vi "RGBtoCMYK.vi"(2 "RGB in":dbl[](array[numeric]), 3 "CMYK in":dbl[](array[numeric])) -> (0 "RGB out":dbl[](array[numeric]), 1 "CMYK out":dbl[](array[numeric]))   [LabVIEW 2013]
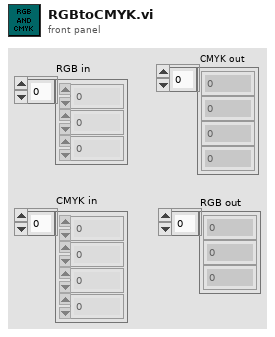
[diagram p1: front panel]
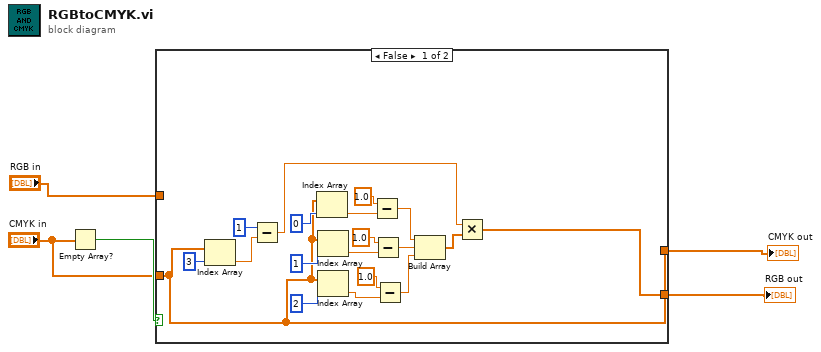
[diagram p0: block diagram]
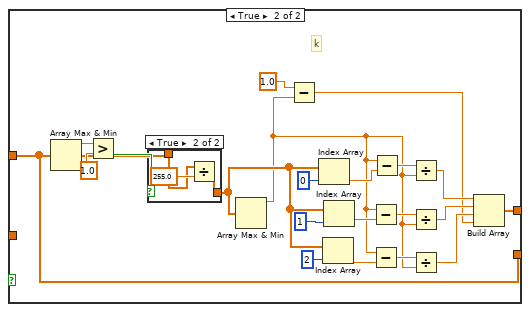
[diagram p2: hidden frame]
diagram:
  n1 = Empty Array?(array="CMYK in") -> (empty?=w4:bool)
  n2 = case shown="False" w4 {
    tunnel: "RGB in" -> [_ w25]
    tunnel: [w18 w26] -> w5
    tunnel: "CMYK in" -> [w18 _]
    tunnel: [w6 w25] -> w1
    frame False {
      n3 = Index Array(array=w18, index=3) -> (element=w23:dbl)
      n4 = Subtract(x=1, y=w23) -> (x-y=w7:dbl)
      n5 = Index Array(array=w18, index=0) -> (element=w14:dbl)
      n6 = Index Array(array=w18, index=1) -> (element=w13:dbl)
      n7 = Index Array(array=w18, index=2) -> (element=w12:dbl)
      n8 = Subtract(x=1.0, y=w14) -> (x-y=w11:dbl)
      n9 = Subtract(x=1.0, y=w13) -> (x-y=w10:dbl)
      n10 = Subtract(x=1.0, y=w12) -> (x-y=w9:dbl)
      n11 = Build Array(w11, w10, w9) -> (w8:dbl[])
      n12 = Multiply(x=w7, y=w8) -> (x*y=w6:dbl[])
    }
    frame True {
      # "k"
      n13 = Array Max & Min(array=w25) -> (max value=w32:dbl)  [unwired: 3 out]
      n14 = Greater?(x=w32, y=1.0) -> (0:w30:bool)
      n15 = case shown="True" w30 {
        tunnel: w25 -> [w46 w48]
        tunnel: [w46 w47] -> w29
        frame False {
        }
        frame True {
          n16 = Divide(x=w48, y=255.0) -> (x/y=w47:dbl[])
        }
      }
      n17 = Array Max & Min(array=w29) -> (max value=w27:dbl)  [unwired: 3 out]
      n18 = Subtract(x=1.0, y=w27) -> (x-y=w33:dbl)
      n19 = Index Array(array=w29, index=0) -> (element=w28:dbl)
      n20 = Index Array(array=w29, index=2) -> (element=w40:dbl)
      n21 = Index Array(array=w29, index=1) -> (element=w41:dbl)
      n22 = Subtract(x=w27, y=w41) -> (x-y=w38:dbl)
      n23 = Subtract(x=w27, y=w40) -> (x-y=w37:dbl)
      n24 = Subtract(x=w27, y=w28) -> (x-y=w39:dbl)
      n25 = Divide(x=w39, y=w27) -> (x/y=w36:dbl)
      n26 = Divide(x=w38, y=w27) -> (x/y=w35:dbl)
      n27 = Divide(x=w37, y=w27) -> (x/y=w34:dbl)
      n28 = Build Array(w36, w35, w34, w33) -> (w26:dbl[])
    }
  }
  "CMYK out" <- w5
  "RGB out" <- w1
